vi "N9310A Set LF Out SR830 Record to file.vi"() -> ()   [LabVIEW 2018]
uses:
  <instrlib>/Stanford Research 830/Public/Data/Read (All Parameters).vi
  <instrlib>/Agilent N9310/Agilent N9310.lvlib
  <instrlib>/Stanford Research 830/Stanford Research 830.lvlib
panel:
  in  "File to save to":path
  out "Measured voltage (V, RMS)":dbl format="%#_6p"
  out "Measured frequency (Hz)":dbl format="%#_6p"
  in  "Input coupling":u16(ring) items=["AC", "DC"]
  in  "Input connection":u16(ring) items=["Single-Ended Voltage", "Differential Voltage", "1 MOhm Current Gain", "100 MOhm Current Gain"]
  in  "Dynamic reserve":i16(ring)=2 items=["High Reserve"=0, "Normal"=1, "Low Noise"=2, "Auto Reserve"=-1]
  in  "Sensitivity":i16(ring)=26 items=["Auto Gain"=-1, "2 nV/fA"=0, "5 nV/fA"=1, "10 nV/fA"=2, "20 nV/fA"=3, "50 nV/fA"=4, "100 nV/fA"=5, "200 nV/fA"=6, "500 nV/fA"=7, "1 uV/pA"=8, "2 uV/pA"=9, "5 uV/pA"=10, "10 uV/pA"=11, "20 uV/pA"=12, "50 uV/pA"=13, "100 uV/pA"=14, "200 uV/pA"=15, "500 uV/pA"=16, "1 mV/nA"=17, "2 mV/nA"=18, "5 mV/nA"=19, "10 mV/nA"=20, "20 mV/nA"=21, "50 mV/nA"=22, "100 mV/nA"=23, "200 mV/nA"=24, "500 mV/mA"=25, "1 V/uA"=26]
  in  "VISA resource name of Stanford SR830":refnum<visa-resource-name>="GPIB0::9::INSTR"
  in  "VISA resource name of Agilent N9310A":refnum<visa-resource-name>="USB0::0x0957::0x2018::01151879::INSTR"
  in  "Wait before measuring (s)":dbl=0.1 format="%#_6p"
  out "Point":dbl format="%^#_6e"
  in  "Points to measure":dbl=10.0 format="%^#_6e"
  in  "Amplitude (V)":dbl=0.5 format="%#_6p"
  in  "Frequency (Hz)":dbl=1000.0 format="%#_6p"
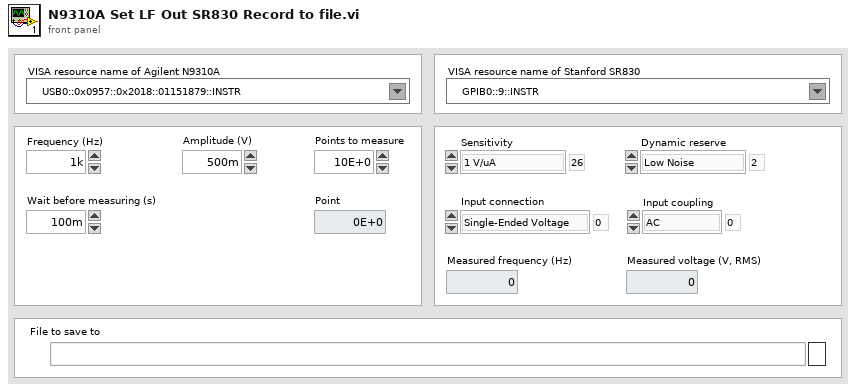
[diagram p1: front panel]
types:
  T1 = cluster{"X-Value":dbl, "Y-Value":dbl, "R-Value":dbl, "Theta-Value":dbl, "Aux In 1 Value":dbl, "Aux In 2 Value":dbl, "Aux In 3 Value":dbl, "Aux In 4 Value":dbl, "Reference Frequency":dbl, "Channel 1 Display":dbl, "Channel 2 Display":dbl}
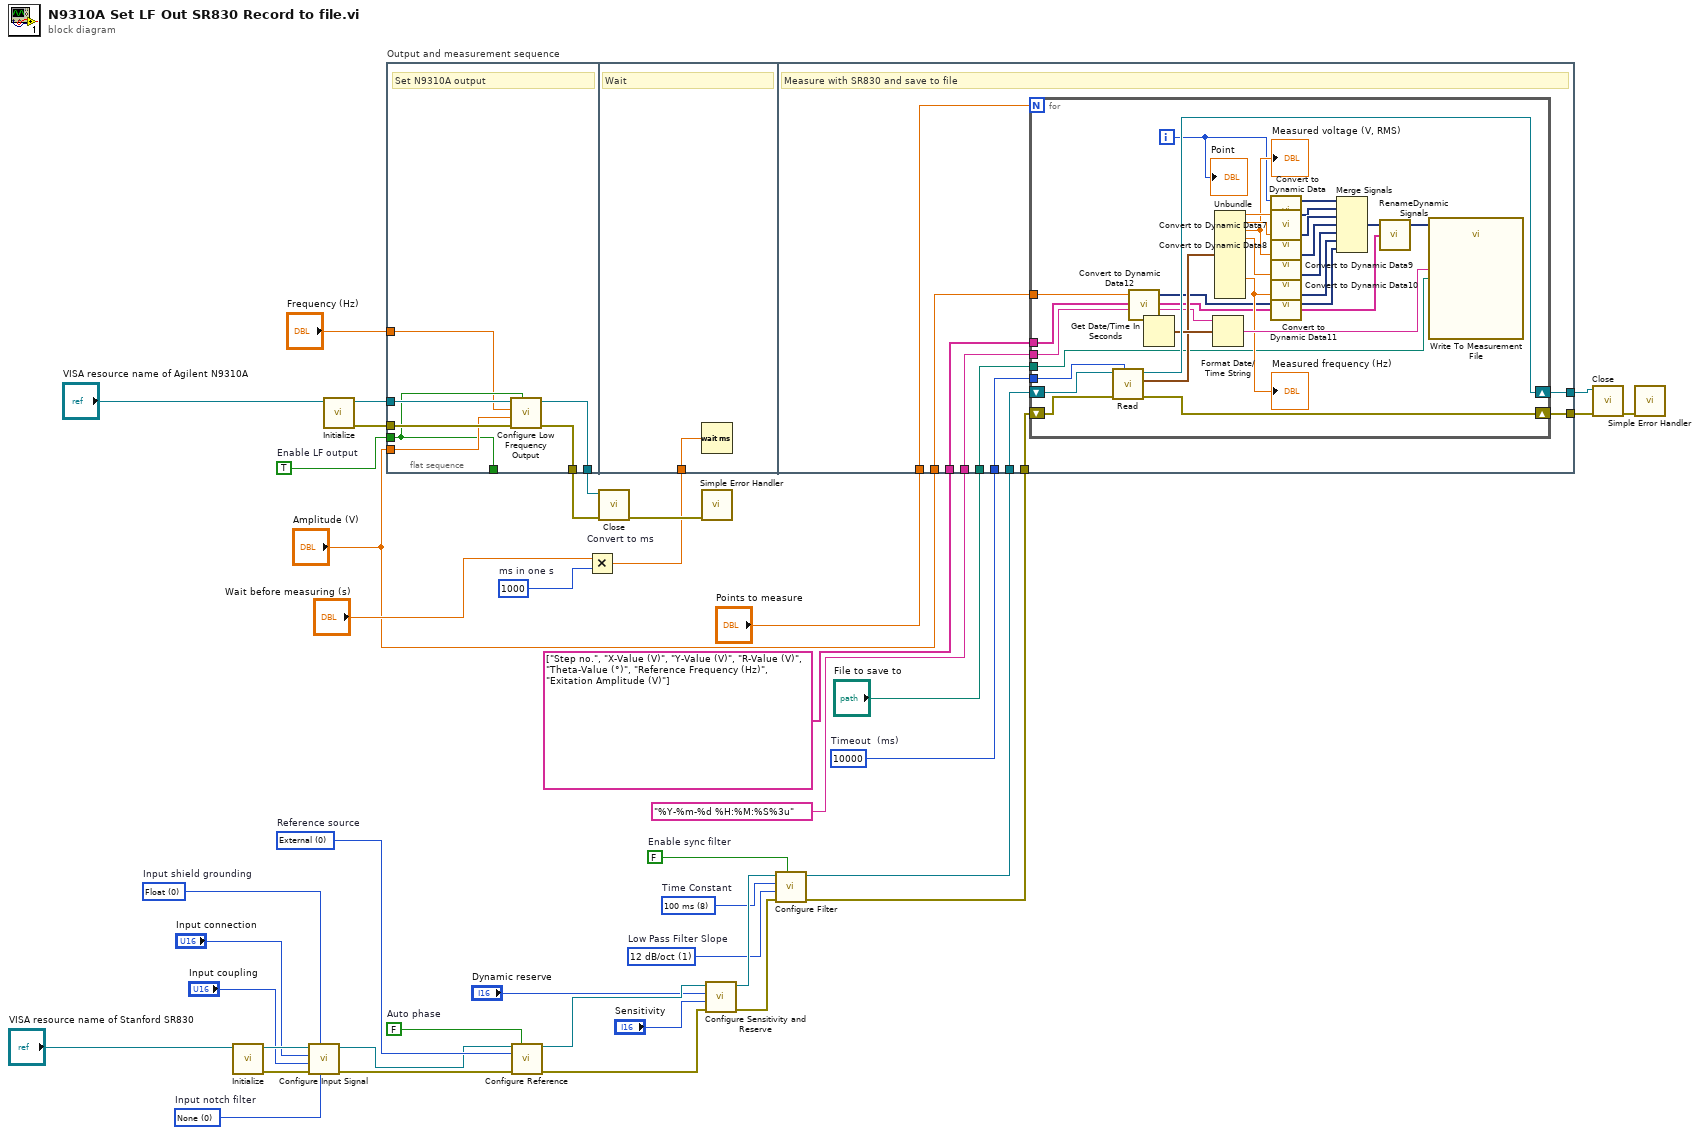
[diagram p0: block diagram]
diagram:
  w6 = u32 10000  # Timeout  (ms)
  w19 = u16 1 items=["6 dB/oct", "12 dB/oct", "18 db/oct", "24 dB/oct"]  # Low Pass Filter Slope
  w20 = u16 8 items=["10 us", "30 us", "100 us", "300 us", "1 ms", "3 ms", "10 ms", "30 ms", "100 ms", "300 ms", "1 s", "3 s", "10 s", "30 s", "100 s", "300 s", "1 ks", "3 ks", "10 ks", "30 ks"]  # Time Constant
  w23 = FALSE  # Enable sync filter
  w28 = FALSE  # Auto phase
  w29 = u16 0 items=["None", "Line Notch", "2x Line Notch", "Both Notch Filters"]  # Input notch filter
  w32 = u16 0 items=["External", "Internal"]  # Reference source
  w36 = u16 0 items=["Float", "Ground"]  # Input shield grounding
  w14 = TRUE  # Enable LF output
  w41 = 1000  # ms in one s
  n1 = call <instrlib>:"Initialize.vi"("VISA resource name"="VISA resource name of Stanford SR830") -> ("error out"=w33:errorcluster, "VISA resource name out"=w37:refnum<visa-resource-name>)  [unwired: 9 in]
  n2 = call <instrlib>:"Configure Input Signal.vi"("Input Notch Filter (0: None)"=w29, "Input Shield Grounding (0: Float)"=w36, "error in (no error)"=w33, "Input Coupling (0: AC)"="Input coupling", "Input Connection (0: Single-Ended Voltage)"="Input connection", "VISA resource name"=w37) -> ("error out"=w30:errorcluster, "VISA resource name out"=w31:refnum<visa-resource-name>)  [unwired: 4 in]
  n3 = call <instrlib>:"Initialize.vi"("VISA resource name"="VISA resource name of Agilent N9310A") -> ("error out"=w15:errorcluster, "VISA resource name out"=w16:refnum<visa-resource-name>)  [unwired: 9 in]
  n4 = flat-sequence "Output and measurement sequence" {
    tunnel: [w46] -> w8
    tunnel: [w45] -> w7
    tunnel: [w44] -> _
    tunnel: w15 -> [w49]
    tunnel: "Amplitude (V)" -> [w48]
    tunnel: w16 -> [w47]
    tunnel: w14 -> [w44]
    tunnel: "Frequency (Hz)" -> [w43]
    tunnel: w17 -> [w50]
    tunnel: [w60] -> w9
    tunnel: [w59] -> w10
    tunnel: w13 -> [w58]
    tunnel: w12 -> [w57]
    tunnel: w6 -> [w56]
    tunnel: "%Y-%m-%d %H:%M:%S%3u" -> [w55]
    tunnel: string[] ["Step no.", "X-Value (V)", "Y-Value (V)", "R-Value (V)", "Theta-Value (°)", "Reference Frequency (Hz)", "Exitation Amplitude (V)"] -> [w54]
    tunnel: "File to save to" -> [w53]
    tunnel: "Points to measure" -> [w52]
    tunnel: "Amplitude (V)" -> [w51]
    frame #0 {
      # "Set N9310A output"
      n5 = call <instrlib>:"Configure Low Frequency Output.vi"("Enable LF Output (F:Disable)"=w44, "error in (no error)"=w49, "Amplitude (0.5 V)"=w48, "Frequency (1.0 kHz)"=w43, "VISA resource name"=w47) -> ("error out"=w46:errorcluster, "VISA resource name out"=w45:refnum<visa-resource-name>)  [unwired: 5 in]
    }
    frame #1 {
      # "Wait"
      n6 = Wait (ms)(milliseconds to wait=w50) -> ()  [unwired: 1 out]
    }
    frame #2 {
      # "Measure with SR830 and save to file"
      n7 = for {
        N: w52 -> [_]
        tunnel: w56 -> [w70]
        tunnel: w55 -> [w69]
        tunnel: w54 -> [w66]
        tunnel: w53 -> [w65]
        shift-right: [w87] -> w60
        shift-left: w58 -> [w72]
        shift-right: [w86] -> w59
        shift-left: w57 -> [w71]
        tunnel: w51 -> [w64]
        i -> [w61]
        n8 = call-poly <instrlib>:"Read.vi"("Timeout (10000 ms)"=w70, "error in (no error)"=w71, "VISA resource name"=w72) -> ("error out"=w86:errorcluster, "Parameter Values"=w74:T1, "VISA resource name out"=w87:refnum<visa-resource-name>)  [unwired: 6 in]
        n9 = call "Convert to Dynamic Data12"("Double"=w64) -> ("Dynamic Data Type"=w63:dynamicdata)  [unwired: 3 in]
        n10 = Get Date/Time In Seconds() -> (seconds since 1Jan1904=w76:timestamp)
        n11 = Format Date/Time String(time format string (%c)=w69, seconds (now)=w76) -> (date/time string=w75:string)  [unwired: 1 in]
        n12 = Unbundle(w74) -> ("X-Value"=w84:dbl, "Y-Value"=w83:dbl, "R-Value"=w67:dbl, "Theta-Value"=w73:dbl, "Reference Frequency"=w68:dbl)  [unwired: 6 out]
        "Measured frequency (Hz)" <- w68
        "Measured voltage (V, RMS)" <- w67
        n13 = call "Convert to Dynamic Data"("Double"=w61) -> ("Dynamic Data Type"=w62:dynamicdata)  [unwired: 3 in]
        n14 = call "Convert to Dynamic Data7"("Double"=w84) -> ("Dynamic Data Type"=w77:dynamicdata)  [unwired: 3 in]
        n15 = call "Convert to Dynamic Data8"("Double"=w83) -> ("Dynamic Data Type"=w78:dynamicdata)  [unwired: 3 in]
        n16 = call "Convert to Dynamic Data9"("Double"=w67) -> ("Dynamic Data Type"=w79:dynamicdata)  [unwired: 3 in]
        n17 = call "Convert to Dynamic Data10"("Double"=w73) -> ("Dynamic Data Type"=w80:dynamicdata)  [unwired: 3 in]
        n18 = call "Convert to Dynamic Data11"("Double"=w68) -> ("Dynamic Data Type"=w81:dynamicdata)  [unwired: 3 in]
        n19 = Merge Signals(w62, w77, w78, w79, w80, w81, w63) -> (w82:dynamicdata)
        n20 = call "RenameDynamicSignals.vi"("New Signal Names"=w66, "Dynamic Data In"=w82) -> ("Dynamic Data Out"=w85:dynamicdata)  [unwired: 2 in, 1 out]
        n21 = call "Write To Measurement File"("Signals"=w85, "Filename"=w65, "Comment"=w75) -> ()  [unwired: 14 in, 3 out]
        "Point" <- w61
      }
    }
  }
  n22 = call <instrlib>:"Configure Reference.vi"("VISA resource name"=w31, "Auto Phase (T: Enabled)"=w28, "Reference Source (1: Internal)"=w32, "error in (no error)"=w30) -> ("VISA resource name out"=w27:refnum<visa-resource-name>, "error out"=w26:errorcluster)  [unwired: 10 in]
  n23 = Multiply "Convert to ms"(x="Wait before measuring (s)", y=w41) -> (x*y=w17:dbl)
  n24 = call <instrlib>:"Close.vi"("error in (no error)"=w8, "VISA resource name"=w7) -> ("error out"=w39:errorcluster)  [unwired: 9 in]
  n25 = call <vilib>:"Simple Error Handler.vi"("error in (no error)"=w39) -> ()  [unwired: 4 in, 5 out]
  n26 = call <instrlib>:"Configure Sensitivity and Reserve.vi"("error in (no error)"=w26, "Sensitivity (-1: Auto gain)"="Sensitivity", "Dynamic Reserve (-1: Auto Reserve)"="Dynamic reserve", "VISA resource name"=w27) -> ("error out"=w21:errorcluster, "VISA resource name out"=w22:refnum<visa-resource-name>)  [unwired: 6 in]
  n27 = call <instrlib>:"Configure Filter.vi"("Enable Sync Filter (F: Disable)"=w23, "error in (no error)"=w21, "Low Pass Filter Slope (1: 12dB/oct)"=w19, "Time Constant (8: 100ms)"=w20, "VISA resource name"=w22) -> ("error out"=w12:errorcluster, "VISA resource name out"=w13:refnum<visa-resource-name>)  [unwired: 5 in]
  n28 = call <instrlib>:"Close.vi"("error in (no error)"=w10, "VISA resource name"=w9) -> ("error out"=w18:errorcluster)  [unwired: 9 in]
  n29 = call <vilib>:"Simple Error Handler.vi"("error in (no error)"=w18) -> ()  [unwired: 4 in, 5 out]
